vi "Read.vi"(8 "error in (no error)":errorcluster, 9 "Timeout (ms)":i32, 10 "Bytes to Read":i32, 11 "IConnection in":refnum<class "IConnection.lvclass">) -> (0 "error out":errorcluster, 1 "TimeOut?":bool, 2 "Data":string, 3 "IConnection out":refnum<class "IConnection.lvclass">)   [LabVIEW 2019, in "Connection Reference.lvlib" / "IConnection.lvclass"]
uses:
  <vilib>/gpm_packages/@cs/Network-interface/Source/Connection Reference/IConnection/IConnection.lvclass
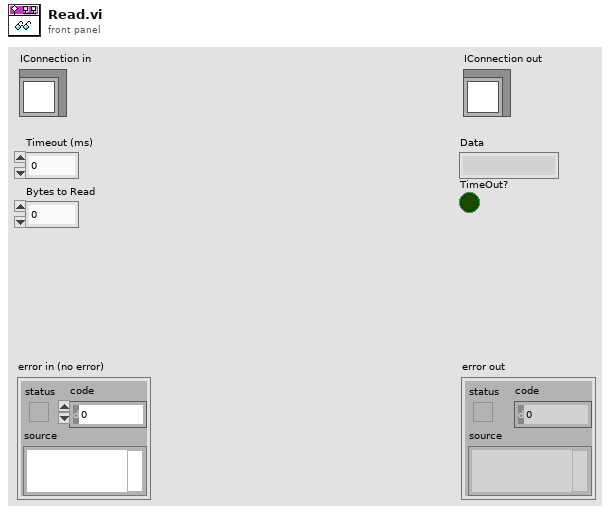
[diagram p1: front panel]
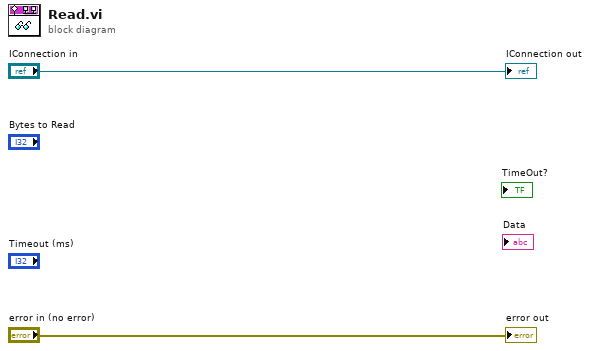
[diagram p0: block diagram]
diagram:
  "error out" <- "error in (no error)"
  "IConnection out" <- "IConnection in"
